vi "UMLEditor Main.vi"(1 "StartProject":string, 3 "StartTarget":string) -> ()   [LabVIEW 2012] (continued)
                              n889 = call-dynamic "translate.vi"("reference"=w2613, "dx"=w2615, "dy"=w2614, "error in (no error)"=w2617) -> ("error out"=w2616:errorcluster)  [unwired: 14 in, 1 out]
                            }
                          }
                        }
                        n890 = Bundle By Name(cluster=w2551, "state"=UMLEditor_statesType."Repaint") -> (w2561:T7)
                        n891 = Array Size(array=w2540) -> (size(s)=w2539:i32)
                        n892 = case shown="Default" w2539 {
                          tunnel: w2559 -> [w2574 w2578]
                          tunnel: [w2574 w2577] -> w2558
                          tunnel: w2553 -> [_ w2576]
                          tunnel: w2540 -> [_ w2575]
                          frame Default {
                          }
                          frame 1.. {
                            n893 = call-dynamic "layout.vi"("reference"=w2576, "LayoutNodes(Empty=All)"=w2575, "error in (no error)"=w2578) -> ("error out"=w2577:errorcluster)  [unwired: 15 in, 1 out]
                          }
                        }
                        n894 = call <resource>:"UMLEditor setDiagramInfo.vi"("error in (no error)"=w2558, "localVariablesIn"=w2561, "action"=enum16{"Name/Dir", "Unsaved", "Saved"}."Unsaved") -> ("localVariablesOut"=w2552:T7, "error out"=w2556:errorcluster)  [unwired: 2 in, 13 out]
                      }
                      frame Default {
                      }
                    }
                  }
                  frame True {
                  }
                }
              }
              frame "Shift" {
                n895 = case shown="Default" w2623 {
                  tunnel: [w2630 w2636] -> w2628
                  tunnel: w2627 -> [w2630 w2635]
                  tunnel: w2626 -> [_ w2634]
                  tunnel: w2625 -> [_ w2633]
                  tunnel: w2624 -> [_ w2632]
                  tunnel: w2622 -> [_ w2631]
                  frame "Key Repeat?" {
                  }
                  frame Default {
                    n896 = case shown="\"Class\"" w2632 {
                      tunnel: [w2637 w2651] -> w2636
                      tunnel: w2635 -> [w2637 w2644]
                      tunnel: w2634 -> [_ w2650]
                      tunnel: w2633 -> [_ w2649]
                      tunnel: w2631 -> [_ w2645]
                      frame "None", Default {
                        # "Only supported in Class Diagram for now"
                      }
                      frame "Class" {
                        n897 = Unbundle By Name(w2649) -> ("zoom"=w2652:dbl, "offset"=w2654:T12)
                        n898 = property on="Picture" class="Pict"() -> ("Mouse"=w2648:T42)  [unwired: 2 in, 2 out]
                        n899 = Unbundle By Name(w2648) -> ("Mouse Position"=w2647:cluster{"X":i32, "Y":i32})
                        n900 = Add(x=w2654, y=w2647) -> (x+y=w2653:T12)
                        n901 = Divide(x=w2653, y=w2652) -> (x/y=w2638:T12)
                        n902 = call <resource>:"UMLEditor_FindObject.vi"("FindManyEdges(False)"=TRUE, "offset"=w2638, "error in"=w2644, "graphics"=w2645, "graph"=w2650) -> ("error out"=w2643:errorcluster, "NodeFound"=w2642:bool, "node"=w2655:refnum<class "AbstractNode.lvclass">, "edge"=w2646:refnum<class "AbstractEdge.lvclass">, "Edges"=w2639:refnum<class "AbstractEdge.lvclass">[], "EdgeFound"=w2641:bool)  [unwired: 1 in]
                        n903 = case shown="False" w2642 {
                          tunnel: [w2658 w2671] -> w2651
                          tunnel: w2655 -> [w2662 w2674]
                          tunnel: w2638 -> [w2661 w2673]
                          tunnel: w2643 -> [w2660 w2672]
                          tunnel: w2641 -> [_ w2670]
                          tunnel: w2646 -> [_ w2669]
                          tunnel: w2639 -> [_ w2668]
                          frame True {
                            n904 = call-dynamic "GetContextHelpInfo.vi"("reference"=w2662, "MousePos"=w2661, "error in (no error)"=w2660) -> ("ContextHelpInfoExist"=w2656:bool, "ContextHelpInfo"=w2657:variant, "error out"=w2659:errorcluster)  [unwired: 13 in, 1 out]
                            n905 = case shown="False" w2656 {
                              tunnel: w2659 -> [w2663 w2667]
                              tunnel: [w2663 w2666] -> w2658
                              tunnel: w2657 -> [_ w2665]
                              frame False {
                              }
                              frame True {
                                n906 = local write "Help"(TRUE ("Help")) -> ()
                                n907 = call <resource>:"ContextHelp_SendMessageToPopUp.vi"("PopUpMessage"=w2665, "error in (no error)"=w2667) -> ("error out"=w2666:errorcluster)  [unwired: 1 in, 16 out]
                              }
                            }
                          }
                          frame False {
                            n908 = case shown="True" w2670 {
                              tunnel: w2674 -> [_ _]
                              tunnel: w2673 -> [_ w2684]
                              tunnel: w2672 -> [w2675 w2687]
                              tunnel: [w2675 w2688] -> w2671
                              tunnel: w2669 -> [_ w2685]
                              tunnel: w2668 -> [_ w2683]
                              frame False {
                              }
                              frame True {
                                w2680 = cluster{string, "empty picture":picture, string} {"Dependencies", "empty picture"=bytes[0], ""}
                                n909 = for {
                                tunnel: w2685 -> [_]
                                tunnel: w2684 -> [w2693]
                                shift-right: [w2694] -> w2686
                                shift-left: w2687 -> [w2695]
                                tunnel: w2683 -> [w2692] mode=indexing
                                tunnel: w2680 -> [_]
                                shift-right: [w2689] -> w2678
                                shift-left: string[] [] -> [w2691]
                                n910 = call-dynamic "GetContextHelpInfo.vi"("reference"=w2692, "MousePos"=w2693, "error in (no error)"=w2695) -> ("Rows"=w2690:string[], "error out"=w2694:errorcluster)  [unwired: 12 in, 3 out]
                                n911 = for {
                                shift-right: [w2699] -> w2689
                                shift-left: w2691 -> [w2698]
                                tunnel: w2690 -> [w2697] mode=indexing
                                n912 = Search 1D Array(1D array=w2698, element=w2697) -> (index of element=w2696:i32)  [unwired: 1 in]
                                n913 = case shown="-1" w2696 {
                                tunnel: w2698 -> [w2700 w2703]
                                tunnel: w2697 -> [_ w2702]
                                tunnel: [w2700 w2701] -> w2699
                                frame Default {
                                }
                                frame -1 {
                                n914 = Build Array (concatenate)(w2703, w2702) -> (w2701:string[])
                                }
                                }
                                }
                                }
                                n915 = Concatenate Strings("<120>", w2678) -> (w2682:string)
                                n916 = Array Size(array=w2678) -> (size(s)=w2677:i32)
                                n917 = Bundle(cluster=w2680, w2682) -> (w2679:cluster{string, "empty picture":picture, string})  [unwired: 2 out]
                                n918 = case shown="0, Default" w2677 {
                                tunnel: w2686 -> [w2704 w2708]
                                tunnel: [w2704 w2707] -> w2688
                                tunnel: w2679 -> [_ w2706]
                                frame 0, Default {
                                }
                                frame 1.. {
                                n919 = local write "Help"(TRUE ("Help")) -> ()
                                n920 = call <resource>:"ContextHelp_SendMessageToPopUp.vi"("PopUpMessage"=w2706, "error in (no error)"=w2708) -> ("error out"=w2707:errorcluster)  [unwired: 1 in, 16 out]
                                }
                                }
                              }
                            }
                          }
                        }
                      }
                    }
                  }
                }
              }
              frame "F5" {
                n921 = Bundle By Name(cluster=w2711, "state"=UMLEditor_statesType."Repaint") -> (w2710:T7)
              }
              frame "Ctrl", "Alt" {
              }
            }
            n922 = event-data() -> ()  [unwired: 1 in, 6 out]
          }
          event Application Instance Close? {
            n923 = event-data() -> ()  [unwired: 3 out]
            n924 = Bundle By Name(cluster=w2718, "state"=UMLEditor_statesType."Exit") -> (w2719:T7)
            n925 = event-data("Discard?"=TRUE) -> ()  [unwired: 1 in, 1 out]
          }
          event Panel Close? {
            w2720 = FALSE ("Sync")
            n926 = event-data() -> ()  [unwired: 4 out]
            n927 = local write "Sync"(w2720) -> ()
            n928 = Bundle By Name(cluster=w2723, "state"=UMLEditor_statesType."Exit", "Sync"=w2720) -> (w2724:T7)
            n929 = event-data("Discard?"=TRUE) -> ()  [unwired: 1 in, 1 out]
          }
          event Menu Selection (User) {
            n930 = event-data() -> ("MenuRef"=w2733:refnum<k9>, "ItemTag"=w2734:string)  [unwired: 5 out]
            n931 = case shown="\"APP_PROJECT_NEW\"" w2734 {
              selector: w2734 -> [w2747 _ _ _ _ _ _ _ _ w2839 _ _ _ _ w2873 w2880 _ _ _ _ w2985 w3045 w3054 w3069 w3085 w3108 _ _ _ _ _ _ _ _ _ _ _ _ _ _]
              tunnel: w2726 -> [w2736 w2760 w2762 w2770 w2786 w2797 w2807 w2813 w2819 w2836 w2852 w2854 w2860 w2866 w2875 w2882 w2885 w2924 w2946 w2954 w2966 w3047 w3057 w3071 w3089 w3111 w3121 w3126 w3128 w3132 w3136 w3140 w3146 w3152 w3161 w3167 w3175 w3178 w3196 w3205]
              tunnel: w2733 -> [_ _ _ _ _ _ _ _ _ w2833 _ _ _ _ _ _ _ _ _ _ _ _ w3062 w3075 _ _ _ _ _ _ _ _ _ _ _ _ _ _ _ _]
              tunnel: w2732 -> [w2748 w2759 w2761 w2767 w2791 w2802 w2804 w2808 w2823 w2830 w2851 w2856 w2862 w2868 w2874 w2884 w2887 w2920 w2950 w2952 w2991 w3049 w3061 w3074 w3088 w3100 w3119 w3123 w3127 w3129 w3133 w3137 w3144 w3150 w3160 w3165 w3174 w3179 w3192 w3206]
              tunnel: [w2748 w2758 w2761 w2763 w2787 w2798 w2804 w2808 w2822 w2841 w2851 w2856 w2862 w2868 w2874 w2884 w2886 w2923 w2950 w2952 w2988 w3049 w3055 w3066 w3087 w3096 w3119 w3123 w3127 w3129 w3133 w3137 w3144 w3150 w3160 w3165 w3173 w3179 w3181 w3206] -> w2731
              tunnel: [w2740 w2760 w2762 w2770 w2785 w2796 w2806 w2813 w2819 w2835 w2852 w2857 w2863 w2869 w2876 w2883 w2885 w2922 w2949 w2953 w2976 w3048 w3056 w3070 w3090 w3112 w3122 w3125 w3128 w3131 w3135 w3139 w3145 w3151 w3161 w3166 w3175 w3177 w3195 w3205] -> w2728
              tunnel: w2730 -> [_ _ _ _ w2790 w2801 _ _ _ _ _ _ _ _ _ _ _ _ _ _ _ _ _ _ _ w3095 _ _ _ _ _ _ _ _ _ _ _ _ w3184 _]
              tunnel: w2729 -> [_ _ _ _ _ _ _ _ _ _ _ _ _ _ _ _ _ _ _ _ _ _ _ _ _ w3094 _ _ _ _ _ _ w3143 w3149 _ w3164 _ _ _ _]
              tunnel: w2727 -> [_ _ _ _ w2783 w2794 _ _ _ _ _ _ _ _ _ _ _ _ _ _ _ _ _ _ _ _ _ _ _ _ _ _ _ _ _ _ _ _ _ _]
              frame Default {
                w2737 = FALSE ("Sync")
                n932 = String To Path(string=w2747) -> (path=w2739:path)
                n933 = Bundle By Name(cluster=w2736, "Sync"=w2737) -> (w2735:T7)
                n934 = local write "Sync"(w2737) -> ()
                n935 = File/Directory Info(path=w2739) -> (directory=w2742:bool, size=w2738:i64, error out=w2745:errorcluster)  [unwired: 1 in, 4 out]
                n936 = To Long Integer(number=w2738) -> (32bit integer=w2746:i32)
                n937 = Unbundle By Name(w2745) -> ("status"=w2743:bool)
                n938 = Greater Than 0?(x=w2746) -> (x > 0?=w2744:bool)
                n939 = Compound Arithmetic op=AND(invert w2742, w2744, invert w2743) -> (w2741:bool)
                n940 = case shown="True" w2741 {
                  tunnel: w2735 -> [w2753 w2757]
                  tunnel: [w2753 w2756] -> w2740
                  tunnel: w2739 -> [w2752 w2754]
                  frame False {
                    n941 = Strip Path(path=w2752) -> (name=w2751:string)  [unwired: 1 out]
                    n942 = Format Into String(format string="File missing\nThis file could not be located.\n%s" ("message"), w2751) -> (resulting string=w2749:string)  [unwired: 2 in, 1 out]
                    n943 = One Button Dialog(message=w2749) -> ()  [unwired: 2 out]
                  }
                  frame True {
                    n944 = Bundle By Name(cluster=w2757, "state"=UMLEditor_statesType."Open", "file"=w2754) -> (w2756:T7)
                  }
                }
              }
              frame "About" {
                n945 = call <resource>:"OpenGDSLicense_ProductInfo.vi"("error in (no error)"=w2759) -> ("error out"=w2758:errorcluster)  [unwired: 18 in]
              }
              frame "APP_PROJECT_NEW" {
                n946 = invoke class="App" method="Project.NewWithPrompts"() -> ()  [unwired: 3 in, 3 out]
              }
              frame "OpenVI" {
                n947 = call "File Dialog2"("prompt"="Select VI to open", "error in"=w2767, "pattern (all files)"="*.vi") -> ("selected path"=w2765:path, "cancelled"=w2764:bool, "error out"=w2766:errorcluster)  [unwired: 4 in, 6 out]
                n948 = case shown="False" w2764 {
                  tunnel: w2766 -> [w2773 w2781]
                  tunnel: w2765 -> [w2772 _]
                  tunnel: [w2771 w2781] -> w2763
                  frame False {
                    n949 = call <resource>:"CommonVIs_UmlOpenVIRef.vi"("error in"=w2773) -> ("error out"=w2775:errorcluster, "AppRefOut"=w2774:refnum<vi>)  [unwired: 3 in, 6 out]
                    n950 = Open VI Reference(application reference (local)=w2774, vi path=w2772, error in (no error)=w2775) -> (vi reference=w2780:refnum<vi>, error out=w2776:errorcluster)  [unwired: 3 out]
                    n951 = property class="VI"(reference=w2780, error in=w2776, "Front Panel Window:Open"=TRUE) -> (reference out=w2778:refnum<vi>, error out=w2777:errorcluster)
                    n952 = Close Reference(reference=w2778, error in (no error)=w2777) -> (error out=w2771:errorcluster)
                  }
                  frame True {
                  }
                }
              }
              frame "Undo" {
                n953 = Unbundle By Name(w2783) -> ("graphics"=w2789:refnum<class "Graphics.lvclass">, "grid"=w2788:refnum<class "Grid.lvclass">)
                n954 = Unbundle By Name(w2783) -> ("menu"=w2782:refnum<k9>)
                n955 = call <resource>:"UndoEngine.vi"("reference"=w2790, "Action"=enum16{"TakeSnapshot", "Undo", "Redo"}."Undo", "graphics"=w2789, "grid"=w2788, "error in (no error)"=w2791, "menu"=w2782) -> ("error out"=w2787:errorcluster)  [unwired: 2 in, 11 out]
                n956 = Bundle By Name(cluster=w2786, "state"=UMLEditor_statesType."Repaint") -> (w2785:T7)
              }
              frame "Redo" {
                n957 = Unbundle By Name(w2794) -> ("graphics"=w2800:refnum<class "Graphics.lvclass">, "grid"=w2799:refnum<class "Grid.lvclass">)
                n958 = Unbundle By Name(w2794) -> ("menu"=w2793:refnum<k9>)
                n959 = call <resource>:"UndoEngine.vi"("reference"=w2801, "Action"=enum16{"TakeSnapshot", "Undo", "Redo"}."Redo", "graphics"=w2800, "grid"=w2799, "error in (no error)"=w2802, "menu"=w2793) -> ("error out"=w2798:errorcluster)  [unwired: 2 in, 11 out]
                n960 = Bundle By Name(cluster=w2797, "state"=UMLEditor_statesType."Repaint") -> (w2796:T7)
              }
              frame "EnterNewLicenceKey" {
                n961 = Bundle By Name(cluster=w2807, "state"=UMLEditor_statesType."CheckLicense") -> (w2806:T7)
              }
              frame "SendComments" {
                n962 = call <resource>:"UMLEditor CommentsDialog.vi"() -> ("nameOut"=w2811:string, "commentsOut"=w2810:string, "canceled"=w2809:bool, "error out"=w2812:errorcluster)  [unwired: 1 in, 15 out]
                n963 = case shown="True" w2809 {
                  tunnel: w2812 -> [w2817 w2818]
                  tunnel: w2811 -> [w2816 _]
                  tunnel: w2810 -> [w2815 _]
                  tunnel: [w2814 w2818] -> _
                  frame False {
                    n964 = call <resource>:"UMLEditor PostComment.vi"("name"=w2816, "comment"=w2815, "error in (no error)"=w2817) -> ("error out"=w2814:errorcluster)  [unwired: 16 out]
                  }
                  frame True {
                  }
                }
              }
              frame "Help_1" {
                n965 = local read "Help"() -> (w2821:bool)
                n966 = Not(x=w2821) -> (.not. x?=w2820:bool)
                n967 = local write "Help"(w2820) -> ()
                n968 = case shown="True" w2820 {
                  tunnel: [ContextHelp_HelpTexts."None(Hide)" ("HelpText") ContextHelp_HelpTexts."Default" ("HelpText")] -> w2824
                  frame False {
                  }
                  frame True {
                  }
                }
                n969 = call <resource>:"ContextHelp_HelpTexts.vi"("HelpText (enum or string)"=w2824) -> ("HelpOut"=w2825:T57)  [unwired: 18 out]
                n970 = call <resource>:"ContextHelp_SendMessageToPopUp.vi"("PopUpMessage"=w2825, "error in (no error)"=w2823) -> ("error out"=w2822:errorcluster)  [unwired: 1 in, 16 out]
              }
              frame "Help_Class Diagram", "Help_Sequence Diagram", "Help_State Diagram", "Help_Use Case Diagram" {
                n971 = local write "Help"("Help") -> ()
                n972 = Set Menu Item Info(6:FALSE ("ToolHelp"), 7:"Show Context Help for tools" ("item tag"), 8:w2830, 11:w2833) -> (0:w2838:errorcluster)  [unwired: 4 out]
                n973 = case shown="True" "Help" {
                  tunnel: [ContextHelp_HelpTexts."None(Hide)" ("HelpText") w2846] -> w2842
                  tunnel: w2839 -> [_ w2845]
                  frame False {
                  }
                  frame True {
                    n974 = case shown="\"Help_Use Case Diagram\"" w2845 {
                      tunnel: [ContextHelp_HelpTexts."ClassDiagram_Help" ("HelpText") ContextHelp_HelpTexts."UseCaseDiagram_Help" ("HelpText") ContextHelp_HelpTexts."SequenceDiagram_Help" ("HelpText") ContextHelp_HelpTexts."StateDiagram_Help" ("HelpText")] -> w2846
                      frame "Help_Class Diagram", Default {
                      }
                      frame "Help_Use Case Diagram" {
                      }
                      frame "Help_Sequence Diagram" {
                      }
                      frame "Help_State Diagram" {
                      }
                    }
                  }
                }
                n975 = call <resource>:"ContextHelp_Memory.vi"("State"=FALSE ("ToolHelp"), "error in (no error)"=w2838, "Actio(GetStatus)n"=T27."SetToolHelp") -> ("error out"=w2831:errorcluster)  [unwired: 1 in, 15 out]
                n976 = call <resource>:"ContextHelp_HelpTexts.vi"("HelpText (enum or string)"=w2842) -> ("HelpOut"=w2843:T57)  [unwired: 18 out]
                n977 = call <resource>:"ContextHelp_SendMessageToPopUp.vi"("PopUpMessage"=w2843, "error in (no error)"=w2831) -> ("error out"=w2841:errorcluster)  [unwired: 1 in, 16 out]
                n978 = Bundle By Name(cluster=w2836, "ToolHelp"=FALSE) -> (w2835:T7)
              }
              frame "GettingStarted" {
                n979 = call <resource>:"UMLEditor GettingStartedDialog.vi"() -> ()  [unwired: 1 out]
              }
              frame "Properties" {
                w2855 = FALSE ("Sync")
                n980 = Bundle By Name(cluster=w2854, "Sync"=w2855) -> (w2853:T7)
                n981 = local write "Sync"(w2855) -> ()
                n982 = Bundle By Name(cluster=w2853, "state"=UMLEditor_statesType."EditSelected") -> (w2857:T7)
              }
              frame "Class Reversed Engineering" {
                w2861 = FALSE ("Sync")
                n983 = Bundle By Name(cluster=w2860, "Sync"=w2861) -> (w2859:T7)
                n984 = local write "Sync"(w2861) -> ()
                n985 = Bundle By Name(cluster=w2859, "state"=UMLEditor_statesType."ClassReversedEngineering") -> (w2863:T7)
              }
              frame "State Reversed Engineering" {
                w2867 = FALSE ("Sync")
                n986 = Bundle By Name(cluster=w2866, "Sync"=w2867) -> (w2865:T7)
                n987 = local write "Sync"(w2867) -> ()
                n988 = Bundle By Name(cluster=w2865, "state"=UMLEditor_statesType."StateReversedEngineering") -> (w2869:T7)
              }
              frame "Delete", "Remove package only" {
                n989 = Equal?(x=w2873, y="Remove package only") -> (x = y?=w2871:bool)
                n990 = Bundle By Name(cluster=w2875, "state"=UMLEditor_statesType."RemoveSelected", "Don'tDeleteChildren"=w2871) -> (w2876:T7)
              }
              frame "Save", "Save As" {
                n991 = Equal?(x="Save As", y=w2880) -> (x = y?=w2878:bool)
                n992 = Bundle By Name(cluster=w2882, "state"=UMLEditor_statesType."Save", "saveAs"=w2878) -> (w2883:T7)
              }
              frame "Export to XMI" {
                (unwired) T58."new or existing file" ("select mode (2)")
                n993 = call <resource>:"UMLEditor getDiagramInfo.vi"("localVariables"=w2885, "error in (no error)"=w2887) -> ("graph"=w2888:refnum<class "Graph.lvclass">, "name"=w2895:string, "diagramType"=w2889:T11, "saveDir"=w2899:path, "error out"=w2890:errorcluster)  [unwired: 13 out]
                n994 = Build Path(base path=w2899, name or relative path=w2895) -> (appended path=w2896:path)
                n995 = call <vilib>:"Get File Extension.vi"("file"=w2896) -> ("filename without extension"=w2897:string)  [unwired: 1 in, 9 out]
                n996 = Concatenate Strings(w2897, ".xmi" ("string")) -> (w2900:string)
                n997 = File Dialog(6:"*.xmi" ("pattern"), 7:"Select file name" ("prompt"), 9:w2900, 11:w2899) -> (1:w2891:bool, 2:w2892:bool, 3:w2902:path)  [unwired: 1 in, 3 out]
                n998 = case shown="True" w2892 {
                  tunnel: [w2910 w2913] -> w2901
                  tunnel: w2891 -> [w2910 _]
                  tunnel: w2902 -> [w2911 w2912]
                  tunnel: [w2911 w2912] -> _
                  frame False {
                  }
                  frame True {
                    n999 = Two Button Dialog(message="This file already exists.\nDo you want to overwrite it?", 1:"No" ("F button name (\"Cancel\")"), 2:"Yes" ("T button name (\"OK\")")) -> (T button?=w2914:bool)
                    n1000 = case shown="True" w2914 {
                      tunnel: w2912 -> [_ w2918]
                      frame False {
                      }
                      frame True {
                        n1001 = Delete(path (use dialog)=w2918) -> ()  [unwired: 1 in, 6 out]
                      }
                    }
                    n1002 = Not(x=w2914) -> (.not. x?=w2913:bool)
                  }
                }
                n1003 = case shown="False" w2901 {
                  tunnel: w2888 -> [w2908 _]
                  tunnel: w2889 -> [w2907 _]
                  tunnel: w2890 -> [w2906 w2909]
                  tunnel: w2902 -> [w2905 _]
                  tunnel: [w2903 w2909] -> w2886
                  frame False {
                    n1004 = call-dynamic "saveGraph.vi"("reference"=w2908, "filePath"=w2905, "diagramType"=w2907, "error in (no error)"=w2906, "ExportType(Normal)"=SaveTypes."XMI") -> ("error out"=w2903:errorcluster)  [unwired: 12 in, 2 out]
                  }
                  frame True {
                  }
                }
              }
              frame "Import from XMI" {
                n1005 = call "File Dialog3"("prompt"="Select XMI file to import", "error in"=w2920, "pattern (all files)"="*.xm?", "pattern label"="XMI file") -> ("selected path"=w2921:path, "exists"=w2927:bool, "cancelled"=w2926:bool, "error out"=w2919:errorcluster)  [unwired: 8 in]
                n1006 = Compound Arithmetic op=AND(w2927, invert w2926, invert w2919) -> (w2925:bool)
                n1007 = case shown="False" w2925 {
                  tunnel: w2924 -> [w2931 w2937]
                  tunnel: w2920 -> [w2932 w2936]
                  tunnel: [w2932 w2936] -> w2923
                  tunnel: [w2931 w2938] -> w2922
                  tunnel: w2921 -> [_ w2935]
                  frame False {
                  }
                  frame True {
                    w2939 = FALSE ("Sync")
                    n1008 = local write "Sync"(w2939) -> ()
                    n1009 = Path To String(path=w2935) -> (string=w2934:string)
                    n1010 = Bundle By Name(cluster=w2937, "selectedEdge"=refnum<class "AbstractEdge.lvclass"> refnum, "SelectedNodes"=refnum<class "AbstractNode.lvclass">[] [], "selcted"=UMLEditor_tooltype."None", "state"=UMLEditor_statesType."ClassReversedEngineering", "toolType"=UMLEditor_tooltype."None", "Sync"=w2939, "Action"=w2934, "XMI_Import"=TRUE ("Sync")) -> (w2938:T7)
                  }
                }
              }
              frame "Open" {
                w2947 = FALSE ("Sync")
                n1011 = Bundle By Name(cluster=w2946, "Sync"=w2947) -> (w2945:T7)
                n1012 = local write "Sync"(w2947) -> ()
                n1013 = Bundle By Name(cluster=w2945, "state"=UMLEditor_statesType."Open") -> (w2949:T7)
              }
              frame "Close" {
                w2951 = FALSE ("Sync")
                n1014 = Unbundle By Name(w2954) -> ("diagrams"=w2961:T39)
                n1015 = Array Size(array=w2961) -> (size(s)=w2960:i32)
                n1016 = Greater Than 0?(x=w2960) -> (x > 0?=w2959:bool)
                n1017 = Select(t=UMLEditor_statesType."Close" ("state"), s=w2959, f=UMLEditor_statesType."Idle" ("state")) -> (s? t:f=w2957:T8)
                n1018 = local write "Sync"(w2951) -> ()
                n1019 = Bundle By Name(cluster=w2954, "state"=w2957, "selcted"=UMLEditor_tooltype."None", "Sync"=w2951) -> (w2953:T7)
              }
              frame "Class Diagram", "Sequence Diagram", "State Diagram", "Use Case Diagram" {
                w2962 = FALSE ("Sync")
                n1020 = case shown="\"State Diagram\"" w2985 {
                  tunnel: w2991 -> [w3027 w3030 w3034 w3038]
                  tunnel: [w3026 w3028 w3032 w3036] -> w2967
                  tunnel: [w3025 w3029 w3033 w3037] -> w2963
                  tunnel: [diagramType."Class" ("diagramType") diagramType."Sequency" ("diagramType") diagramType."UseCase" ("diagramType") diagramType."State" ("diagramType")] -> w2978
                  frame "Class Diagram", Default {
                    n1021 = call <resource>:"ClassDiagramGraph_Create.vi"("error in (no error)"=w3027) -> ("reference out"=w3026:refnum<class "ClassDiagramGraph.lvclass">, "error out"=w3025:errorcluster)  [unwired: 2 in, 15 out]
                  }
                  frame "Sequence Diagram" {
                    n1022 = call <resource>:"SequenceDiagramGraph_Create.vi"("error in (no error)"=w3030) -> ("reference out"=w3028:refnum<class "SequenceDiagramGraph.lvclass">, "error out"=w3029:errorcluster)  [unwired: 2 in, 15 out]
                  }
                  frame "Use Case Diagram" {
                    n1023 = call <resource>:"UseCaseDiagramGraph_Create.vi"("error in (no error)"=w3034) -> ("reference out"=w3032:refnum<class "UseCaseDiagramGraph.lvclass">, "error out"=w3033:errorcluster)  [unwired: 2 in, 15 out]
                  }
                  frame "State Diagram" {
                    n1024 = call <resource>:"StateDiagramGraph_Create.vi"("error in (no error)"=w3038) -> ("reference out"=w3036:refnum<class "StateDiagramGraph.lvclass">, "error out"=w3037:errorcluster)  [unwired: 3 in, 14 out]
                  }
                }
                n1025 = property on="toolTab" class="TabCtl (strict)"("Disabled"=u8 0) -> ()  [unwired: 2 in, 2 out]
                n1026 = local write "Diagram"(0) -> ()
                n1027 = property on="Picture" class="Pict"("Visible"=TRUE) -> ()  [unwired: 2 in, 2 out]
                n1028 = Unbundle By Name(w2966) -> ("diagrams"=w2996:T39)
                n1029 = Unbundle By Name(w2966) -> ("menu"=w2965:refnum<k9>)
                n1030 = for {
                  tunnel: w2996 -> [w3043] mode=indexing
                  tunnel: "Untitled %d" -> [w3041]
                  tunnel: [w3040] -> w2994 mode=indexing
                  n1031 = Unbundle By Name(w3043) -> ("name"=w3042:string)
                  n1032 = Scan From String(format string=w3041, input string=w3042) -> (output 1=w3040:i32)  [unwired: 2 in, 4 out]
                }
                n1033 = call <resource>:"UndoEngine.vi"("reference"=w2967, "Action"=enum16{"TakeSnapshot", "Undo", "Redo"}."TakeSnapshot", "Reset"=TRUE, "error in (no error)"=w2963, "menu"=w2965) -> ("error out"=w2964:errorcluster)  [unwired: 3 in, 11 out]
                n1034 = local read "Help"() -> (w2979:bool)
                n1035 = Array Max & Min(array=w2994) -> (max value=w2993:i32)  [unwired: 3 out]
                n1036 = case shown="True" w2979 {
                  tunnel: w2978 -> [_ w3000]
                  frame False {
                  }
                  frame True {
                    n1037 = case shown="\"Class\", Default" w3000 {
                      tunnel: [ContextHelp_HelpTexts."ClassDiagram_Help" ("HelpText") ContextHelp_HelpTexts."UseCaseDiagram_Help" ("HelpText") ContextHelp_HelpTexts."SequenceDiagram_Help" ("HelpText") ContextHelp_HelpTexts."StateDiagram_Help" ("HelpText")] -> w2998
                      frame "Class", Default {
                      }
                      frame "UseCase" {
                      }
                      frame "Sequency" {
                      }
                      frame "State" {
                      }
                    }
                    n1038 = call <resource>:"ContextHelp_HelpTexts.vi"("HelpText (enum or string)"=w2998) -> ("HelpOut"=w2999:T57)  [unwired: 18 out]
                    n1039 = call <resource>:"ContextHelp_SendMessageToPopUp.vi"("PopUpMessage"=w2999) -> ()  [unwired: 2 in, 17 out]
                  }
                }
                n1040 = Increment(x=w2993) -> (x+1=w2990:i32)
                n1041 = call <resource>:"UMLEditor UpdatesToolbuttons.vi"() -> ()  [unwired: 6 in, 14 out]
                n1042 = Format Into String(format string="Untitled %d", w2990) -> (resulting string=w2982:string)  [unwired: 2 in, 1 out]
                n1043 = call <resource>:"UMLEditor addDiagram.vi"("graph"=w2967, "diagramType"=w2978, "name"=w2982, "saveDir"=path "", "unsaved(False)"=FALSE, "error in (no error)"=w2964, "localVariablesIn"=w2966) -> ("localVariablesOut"=w2983:T7, "error out"=w2987:errorcluster)  [unwired: 11 out]
                n1044 = property on="Diagram" class="Ring (strict)"("Tip Strip"=w2982) -> ()  [unwired: 2 in, 2 out]
                n1045 = case shown="\"Sequency\"" w2978 {
                  tunnel: w2983 -> [w3006 w3010 w3014 w3019 w3023]
                  tunnel: [w3005 w3009 w3013 w3018 w3022] -> w2975
                  frame "None" {
                    n1046 = Bundle By Name(cluster=w3006, "tool"=UMLEditor_toolsType."CD_Select") -> (w3005:T7)
                  }
                  frame "Sequency" {
                    n1047 = Bundle By Name(cluster=w3010, "tool"=UMLEditor_toolsType."SQD_Select") -> (w3009:T7)
                    n1048 = property on="toolTab" class="TabCtl (strict)"("Value"=enum32{"Class", "Sequence", "UseCase"}."Sequence" ("toolTab")) -> ()  [unwired: 2 in, 2 out]
                  }
                  frame "UseCase" {
                    n1049 = Bundle By Name(cluster=w3014, "tool"=UMLEditor_toolsType."UD_Select") -> (w3013:T7)
                    n1050 = property on="toolTab" class="TabCtl (strict)"("Value"=enum32{"Class", "Sequence", "UseCase"}."UseCase" ("toolTab")) -> ()  [unwired: 2 in, 2 out]
                  }
                  frame "State" {
                    n1051 = Bundle By Name(cluster=w3019, "tool"=UMLEditor_toolsType."STD_Select") -> (w3018:T7)
                    n1052 = property on="toolTab" class="TabCtl (strict)"("Value"=enum32{"Class", "Sequence", "UseCase", "State"}."State" ("toolTab")) -> ()  [unwired: 2 in, 2 out]
                  }
                  frame "Class", Default {
                    n1053 = Bundle By Name(cluster=w3023, "tool"=UMLEditor_toolsType."CD_Select") -> (w3022:T7)
                    n1054 = property on="toolTab" class="TabCtl (strict)"("Value"=enum32{"Class", "Sequence", "UseCase"}."Class" ("toolTab")) -> ()  [unwired: 2 in, 2 out]
                  }
                }
                n1055 = Unbundle By Name(w2966) -> ("menu"=w2977:refnum<k9>)
                n1056 = Bundle By Name(cluster=w2975, "selectedEdge"=refnum<class "AbstractEdge.lvclass"> refnum, "SelectedNodes"=refnum<class "AbstractNode.lvclass">[] [], "selcted"=UMLEditor_tooltype."None", "state"=UMLEditor_statesType."Repaint", "toolType"=UMLEditor_tooltype."None", "Sync"=w2962) -> (w2976:T7)
                n1057 = local write "Sync"(w2962) -> ()
                n1058 = call <resource>:"UMLEditor menuUpdates.vi"("menu"=w2977, "menuAction"=UMLEditor_MenuActionType."EnableSave", "error in (no error)"=w2987) -> ("error out"=w2988:errorcluster)  [unwired: 3 in, 13 out]
              }
              frame "Print", "jpg", "png" {
                n1059 = case shown="\"Print\", Default" w3045 {
                  tunnel: [UMLEditor_ExportType."Printer" ("exportype") UMLEditor_ExportType."png" ("exportype") UMLEditor_ExportType."jpg" ("exportype")] -> w3044
                  frame "Print", Default {
                  }
                  frame "png" {
                  }
                  frame "jpg" {
                  }
                }
                n1060 = Bundle By Name(cluster=w3047, "state"=UMLEditor_statesType."Export", "exportype"=w3044) -> (w3048:T7)
              }
              frame "Hide Grid" {
                n1061 = Get Menu Item Info(7:w3054, 8:w3061, 11:w3062) -> (0:w3060:errorcluster, 3:w3053:refnum<k9>, 4:w3059:bool)  [unwired: 4 out]
                n1062 = Not(x=w3059) -> (.not. x?=w3058:bool)
                n1063 = Set Menu Item Info(6:w3058, 7:w3054, 8:w3060, 11:w3053) -> (0:w3055:errorcluster)  [unwired: 4 out]
                n1064 = Bundle By Name(cluster=w3057, "state"=UMLEditor_statesType."Repaint", "hideGrid"=w3058) -> (w3056:T7)
              }
              frame "Show Context Help for tools" {
                n1065 = Get Menu Item Info(7:w3069, 8:w3074, 11:w3075) -> (0:w3073:errorcluster, 3:w3068:refnum<k9>, 4:w3072:bool)  [unwired: 4 out]
                n1066 = Not(x=w3072) -> (.not. x?=w3064:bool)
                n1067 = Set Menu Item Info(6:w3064, 7:w3069, 8:w3073, 11:w3068) -> (0:w3067:errorcluster)  [unwired: 4 out]
                n1068 = call <resource>:"ContextHelp_Memory.vi"("State"=w3064, "error in (no error)"=w3067, "Actio(GetStatus)n"=T27."SetToolHelp") -> ("error out"=w3066:errorcluster)  [unwired: 1 in, 15 out]
                n1069 = Bundle By Name(cluster=w3071, "ToolHelp"=w3064) -> (w3070:T7)
              }
              frame "Zoom In", "Zoom Out" {
                w3080 = 1.5 ("x")
                n1070 = Unbundle By Name(w3089) -> ("graphics"=w3091:refnum<class "Graphics.lvclass">, "zoom"=w3086:dbl)
                n1071 = Equal?(x=w3085, y="Zoom In") -> (x = y?=w3082:bool)
                n1072 = Square Root(x=w3080) -> ()  [unwired: 1 out]
                n1073 = Multiply(x=w3086, y=w3080) -> (x*y=w3083:dbl)
                n1074 = Divide(x=w3086, y=w3080) -> (x/y=w3081:dbl)
                n1075 = Select(t=w3083, s=w3082, f=w3081) -> (s? t:f=w3077:dbl)
                n1076 = In Range and Coerce(upper limit=5.0625, x=w3077, lower limit=0.197530864) -> (coerced(x)=w3076:dbl)  [unwired: 1 out]
                n1077 = call <resource>:"scale.vi"("reference"=w3091, "scaleX"=w3076, "scaleY"=w3076, "error in (no error)"=w3088) -> ("error out"=w3087:errorcluster)  [unwired: 15 out]
                n1078 = Bundle By Name(cluster=w3089, "zoom"=w3076, "state"=UMLEditor_statesType."Repaint") -> (w3090:T7)
              }
              frame "Larger Grid", "Smaller Grid" {
                n1079 = Unbundle By Name(w3111) -> ("grid"=w3099:refnum<class "Grid.lvclass">, "gridSize"=w3110:dbl)
                n1080 = Equal?(x=w3108, y="Larger Grid") -> (x = y?=w3105:bool)
                n1081 = Square Root(x=2.0) -> (sqrt(x)=w3109:dbl)
                n1082 = Multiply(x=w3110, y=w3109) -> (x*y=w3106:dbl)
                n1083 = Divide(x=w3110, y=w3109) -> (x/y=w3104:dbl)
                n1084 = call <resource>:"ForceUpdate.vi"("Set"=TRUE) -> ()  [unwired: 18 in, 1 out]
                n1085 = Select(t=w3106, s=w3105, f=w3104) -> (s? t:f=w3103:dbl)
                n1086 = In Range and Coerce(upper limit=100.0, x=w3103, lower limit=4.0) -> (coerced(x)=w3098:dbl)  [unwired: 1 out]
                n1087 = call <resource>:"setGrid.vi"("reference"=w3099, "gridX"=w3098, "gridY"=w3098, "error in (no error)"=w3100) -> ("error out"=w3097:errorcluster)  [unwired: 15 out]
                n1088 = case shown="Default" w3094 {
                  tunnel: w3097 -> [w3117 w3118]
                  tunnel: [w3116 w3118] -> w3096
                  tunnel: w3095 -> [w3115 _]
                  frame Default {
                    n1089 = call-dynamic "layout.vi"("reference"=w3115, "error in (no error)"=w3117) -> ("error out"=w3116:errorcluster)  [unwired: 16 in, 1 out]
                  }
                  frame "None" {
                  }
                }
                n1090 = Bundle By Name(cluster=w3111, "gridSize"=w3098, "state"=UMLEditor_statesType."Repaint") -> (w3112:T7)
              }
              frame "Exit" {
                n1091 = Bundle By Name(cluster=w3121, "state"=UMLEditor_statesType."Exit") -> (w3122:T7)
              }
              frame "createScript" {
                n1092 = Bundle By Name(cluster=w3126, "state"=UMLEditor_statesType."CreateScript") -> (w3125:T7)
              }
              frame "Open GOOP Wizard" {
                n1093 = call <resource>:"UMLEditor SendMessageToWizard.vi"("error in (no error)"=w3127) -> ()  [unwired: 3 in, 16 out]
              }
              frame "executeScript" {
                n1094 = Bundle By Name(cluster=w3132, "state"=UMLEditor_statesType."ExecuteScript") -> (w3131:T7)
              }
              frame "Copy Selected Nodes" {
                n1095 = Bundle By Name(cluster=w3136, "state"=UMLEditor_statesType."Copy") -> (w3135:T7)
              }
              frame "Paste Nodes" {
                n1096 = Bundle By Name(cluster=w3140, "state"=UMLEditor_statesType."Paste") -> (w3139:T7)
              }
              frame "AutoPlace" {
                n1097 = Not Equal?(x=diagramType."Class", y=w3143) -> ()  [unwired: 1 out]
                n1098 = Bundle By Name(cluster=w3146, "state"=UMLEditor_statesType."AutoPlace") -> (w3145:T7)
              }
              frame "Synchronize All" {
                n1099 = Not Equal?(x=diagramType."Class", y=w3149) -> (x != y?=w3147:bool)
                n1100 = case shown="False" w3147 {
                  tunnel: w3152 -> [w3155 w3157]
                  tunnel: [w3154 w3157] -> w3151
                  frame False {
                    n1101 = Bundle By Name(cluster=w3155, "state"=UMLEditor_statesType."SyncAll") -> (w3154:T7)
                  }
                  frame True {
                    n1102 = One Button Dialog(message="This is only valid for Class Diagrams") -> ()  [unwired: 2 out]
                  }
                }
              }
              frame "ToggleSync" {
                n1103 = property on="Sync" class="Bool (strict)"() -> ("Value"=w3158:bool)  [unwired: 2 in, 2 out]
                n1104 = Not(x=w3158) -> (.not. x?=w3159:bool)
                n1105 = property on="Sync" class="Bool (strict)"("Val(Sgnl)"=w3159) -> ()  [unwired: 2 in, 2 out]
              }
              frame "StraightenAssociations" {
                n1106 = Not Equal?(x=diagramType."Class", y=w3164) -> (x != y?=w3162:bool)
                n1107 = case shown="False" w3162 {
                  tunnel: w3167 -> [w3170 w3172]
                  tunnel: [w3169 w3172] -> w3166
                  frame False {
                    n1108 = Bundle By Name(cluster=w3170, "state"=UMLEditor_statesType."StraightenAssociation") -> (w3169:T7)
                  }
                  frame True {
                    n1109 = One Button Dialog(message="This is only valid for Class Diagrams") -> ()  [unwired: 2 out]
                  }
                }
              }
              frame "Revision history" {
                n1110 = call <resource>:"UMLEditor RevisionHistory.vi"("localVariables"=w3175, "error in (no error)"=w3174) -> ("error out"=w3173:errorcluster)  [unwired: 17 out]
              }
              frame "PlugInRev" {
                n1111 = Bundle By Name(cluster=w3178, "state"=UMLEditor_statesType."PlugInReverseEngineering") -> (w3177:T7)
              }
              frame "Options" {
                n1112 = call <resource>:"GetUndoOption.vi"("error in (no error)"=w3192) -> ("UndoSize"=w3189:i32, "error out"=w3191:errorcluster)  [unwired: 17 out]
                n1113 = call <resource>:"UMLEditor_OptionsDialog.vi"("localVariables"=w3196, "error in (no error)"=w3191) -> ("error out"=w3190:errorcluster)  [unwired: 1 in, 16 out]
                n1114 = call <resource>:"GetUndoOption.vi"("error in (no error)"=w3190) -> ("UndoSize"=w3183:i32, "error out"=w3187:errorcluster)  [unwired: 17 out]
                n1115 = Unbundle By Name(w3196) -> ("menu"=w3185:refnum<k9>)
                n1116 = Not Equal?(x=w3183, y=w3189) -> (x != y?=w3188:bool)
                n1117 = case shown="True" w3188 {
                  tunnel: w3187 -> [w3197 w3204]
                  tunnel: [w3197 w3203] -> w3186
                  tunnel: w3185 -> [_ w3200]
                  tunnel: w3184 -> [_ w3199]
                  tunnel: w3183 -> [_ w3198]
                  frame False {
                  }
                  frame True {
                    n1118 = call <resource>:"UndoEngine.vi"("reference"=w3199, "Action"=enum16{"TakeSnapshot", "Undo", "Redo"}."TakeSnapshot", "Reset"=TRUE, "error in (no error)"=w3204, "menu"=w3200, "UndoLevels(ignoredIfNotWired)"=w3198) -> ("error out"=w3203:errorcluster)  [unwired: 2 in, 11 out]
                  }
                }
                n1119 = call <resource>:"UMLEditor AddToolsMenuItems.vi"("menu"=w3185, "GoopWizExists"=FALSE, "error in (no error)"=w3186) -> ("error out"=w3182:errorcluster)  [unwired: 1 in, 15 out]
                n1120 = call <resource>:"GetSyncOption.vi"("error in (no error)"=w3182) -> ("SyncTime(s)"=w3180:i32, "error out"=w3181:errorcluster)  [unwired: 16 in, 1 out]
                n1121 = Bundle By Name(cluster=w3196, "state"=UMLEditor_statesType."Repaint", "SyncTime"=w3180) -> (w3195:T7)
              }
              frame "ShowTips" {
                n1122 = call <resource>:"ShowToolTips.vi"() -> ()  [unwired: 1 in, 19 out]
              }
            }
          }
          event "open": Value Change {
            n1123 = event-data() -> ()  [unwired: 6 out]
            n1124 = Bundle By Name(cluster=w3208, "state"=UMLEditor_statesType."Open") -> (w3209:T7)
          }
          event "Sync": Value Change {
            n1125 = event-data() -> ()  [unwired: 2 out]
            n1126 = case shown="False" "Sync" {
              selector: "Sync" -> [_ w3218]
              tunnel: [FALSE w3220] -> w3211
              tunnel: w3213 -> [_ w3219]
              frame False {
                n1127 = local write "StatusBar"("" ("StatusBar")) -> ()
              }
              frame True {
                n1128 = call <resource>:"UMLEditor getDiagramInfo.vi"("localVariables"=w3219) -> ("graph"=w3221:refnum<class "Graph.lvclass">, "diagramType"=w3222:T11)  [unwired: 1 in, 16 out]
                n1129 = case shown="\"Class\"" w3222 {
                  tunnel: w3218 -> [_ _]
                  tunnel: w3221 -> [_ w3232]
                  tunnel: [FALSE w3230] -> w3220
                  frame "None", Default {
                    n1130 = One Button Dialog(message="Only class diagrams can have auto synchronization turn on.") -> ()  [unwired: 1 in, 1 out]
                  }
                  frame "Class" {
                    n1131 = call-dynamic "getNodes.vi"("reference"=w3232) -> ("nodes"=w3229:refnum<class "AbstractNode.lvclass">[])  [unwired: 16 in, 2 out]
                    n1132 = for {
                      tunnel: w3229 -> [w3239] mode=indexing
                      tunnel: [w3235] -> w3231
                      stop <- w3235 continue-if-true
                      w3238 = refnum<class "ClassNode.lvclass"> refnum  # ClassNode.lvclass
                      n1133 = To More Specific Class(target class=w3238, reference=w3239) -> (specific class reference=w3237:refnum<class "ClassNode.lvclass">, error out=w3236:errorcluster)  [unwired: 1 in]
                      n1134 = case shown="No Error" w3236 {
                        selector: w3236 -> [w3245 w3247]
                        tunnel: w3237 -> [w3246 _]
                        tunnel: [w3241 w3247] -> w3235
                        frame No Error {
                          n1135 = call-dynamic "getClassInfo.vi"("reference"=w3246, "error in (no error)"=w3245) -> ("className"=w3242:string)  [unwired: 8 in, 9 out]
                          n1136 = Format Into String(format string="%s.lvclass:%s.ctl", w3242, w3242) -> (resulting string=w3243:string)  [unwired: 2 in, 1 out]
                          n1137 = call <resource>:"CommonVIs_UmlOpenVIRef.vi"("ViPath/ViName"=w3243) -> ("error out"=w3241:errorcluster, "vi reference"=w3240:refnum<vi>)  [unwired: 3 in, 6 out]
                          n1138 = Close Reference(reference=w3240) -> ()  [unwired: 1 in, 1 out]
                        }
                        frame Error {
                        }
                      }
                    }
                    n1139 = Array Size(array=w3229) -> (size(s)=w3228:i32)
                    n1140 = Equal To 0?(x=w3228) -> (x = 0?=w3226:bool)
                    n1141 = Unbundle(w3231) -> ("status"=w3227:bool)  [unwired: 2 out]
                    n1142 = Or(x=w3227, y=w3226) -> (x .or. y?=w3225:bool)
                    n1143 = case shown="True" w3225 {
                      tunnel: [TRUE _] -> w3230
                      frame False {
                      }
                      frame True {
                        n1144 = One Button Dialog(message="Synchronization can't be turned on for this diagram. Make sure at least one class have a class path defined and that the classes are in memory.") -> ()  [unwired: 1 in, 1 out]
                      }
                    }
                  }
                }
              }
            }
            n1145 = Bundle By Name(cluster=w3213, "ForceSyncNow"=w3211, "Sync"=w3211) -> (w3214:T7)
            n1146 = local write "Sync"(w3211) -> ()
          }
          event "close": Value Change {
            n1147 = event-data() -> ()  [unwired: 6 out]
            n1148 = Unbundle By Name(w3256) -> ("diagrams"=w3255:T39)
            n1149 = Array Size(array=w3255) -> (size(s)=w3254:i32)
            n1150 = Greater Than 0?(x=w3254) -> (x > 0?=w3253:bool)
            n1151 = Select(t=UMLEditor_statesType."Close" ("state"), s=w3253, f=UMLEditor_statesType."Idle" ("state")) -> (s? t:f=w3251:T8)
            n1152 = Bundle By Name(cluster=w3256, "state"=w3251, "selcted"=UMLEditor_tooltype."None") -> (w3257:T7)
          }
          event "Diagram": Value Change {
            n1153 = event-data() -> ()  [unwired: 2 out]
            n1154 = call <resource>:"UMLEditor UpdatesToolbuttons.vi"() -> ()  [unwired: 6 in, 14 out]
            n1155 = Bundle By Name(cluster=w3279, "state"=UMLEditor_statesType."Repaint", "diagramIndex"="Diagram", "toolType"=UMLEditor_tooltype."None", "selectedEdge"=refnum<class "AbstractEdge.lvclass"> refnum, "SelectedNodes"=refnum<class "AbstractNode.lvclass">[] []) -> (w3259:T7)
            n1156 = Unbundle By Name(w3259) -> ("menu"=w3258:refnum<k9>)
            n1157 = call <resource>:"UMLEditor getDiagramInfo.vi"("localVariables"=w3259, "error in (no error)"=w3276) -> ("graph"=w3262:refnum<class "Graph.lvclass">, "name"=w3267:string, "diagramType"=w3275:T11, "saveDir"=w3270:path, "error out"=w3261:errorcluster)  [unwired: 13 out]
            n1158 = case shown="\"Class\", Default" w3275 {
              tunnel: w3259 -> [w3284 w3288 w3292 w3296 w3301]
              tunnel: [w3283 w3287 w3291 w3295 w3300] -> w3274
              frame "None" {
                n1159 = property on="toolTab" class="TabCtl (strict)"("Disabled"=u8 2) -> ()  [unwired: 2 in, 2 out]
                n1160 = Bundle By Name(cluster=w3284, "tool"=UMLEditor_toolsType."CD_Select") -> (w3283:T7)
              }
              frame "Sequency" {
                n1161 = property on="toolTab" class="TabCtl (strict)"("Value"=enum32{"Class", "Sequence", "UseCase"}."Sequence" ("toolTab")) -> ()  [unwired: 2 in, 2 out]
                n1162 = Bundle By Name(cluster=w3288, "tool"=UMLEditor_toolsType."SQD_Select") -> (w3287:T7)
              }
              frame "State" {
                n1163 = Bundle By Name(cluster=w3292, "tool"=UMLEditor_toolsType."STD_Select") -> (w3291:T7)
                n1164 = property on="toolTab" class="TabCtl (strict)"("Value"=enum32{"Class", "Sequence", "UseCase", "State"}."State" ("toolTab")) -> ()  [unwired: 2 in, 2 out]
              }
              frame "UseCase" {
                n1165 = property on="toolTab" class="TabCtl (strict)"("Value"=enum32{"Class", "Sequence", "UseCase"}."UseCase" ("toolTab")) -> ()  [unwired: 2 in, 2 out]
                n1166 = Bundle By Name(cluster=w3296, "tool"=UMLEditor_toolsType."UD_Select") -> (w3295:T7)
              }
              frame "Class", Default {
                n1167 = property on="toolTab" class="TabCtl (strict)"("Value"=enum32{"Class", "Sequence", "UseCase"}."Class" ("toolTab")) -> ()  [unwired: 2 in, 2 out]
                n1168 = Bundle By Name(cluster=w3301, "tool"=UMLEditor_toolsType."CD_Select") -> (w3300:T7)
              }
            }
            n1169 = Empty String/Path?(string/path=w3270) -> (empty?=w3269:bool)
            n1170 = Build Path(base path=w3270, name or relative path=w3267) -> (appended path=w3272:path)
            n1171 = call <resource>:"UndoEngine.vi"("reference"=w3262, "Action"=enum16{"TakeSnapshot", "Undo", "Redo"}."TakeSnapshot", "Reset"=TRUE, "error in (no error)"=w3261, "menu"=w3258) -> ("error out"=w3260:errorcluster)  [unwired: 3 in, 11 out]
            n1172 = Path To String(path=w3272) -> (string=w3271:string)
            n1173 = case shown="False" w3269 {
              tunnel: w3271 -> [w3280 _]
              tunnel: [w3280 w3281] -> w3268
              tunnel: w3267 -> [_ w3281]
              frame False {
              }
              frame True {
              }
            }
            n1174 = property on="Diagram" class="Ring (strict)"("Tip Strip"=w3268) -> ()  [unwired: 2 in, 2 out]
          }
          event Panel Resize {
            w3302 = FALSE ("Sync")
            n1175 = event-data() -> ()  [unwired: 9 out]
            n1176 = local write "Sync"(w3302) -> ()
            n1177 = Bundle By Name(cluster=w3305, "ResizePanelInProgress"=TRUE, "Sync"=w3302) -> (w3304:T7)
          }
          event "Picture": Mouse Leave {
            n1178 = event-data() -> ()  [unwired: 5 out]
            n1179 = Unbundle By Name(w3313) -> ("butDwn"=w3312:bool)
            n1180 = call-poly <vilib>:"Set Cursor.vi"("VI reference (current VI)"=w3307, "icon"=u16 0) -> ()  [unwired: 1 in, 9 out]
            n1181 = Select(t=UMLEditor_statesType."Repaint" ("state"), s=w3312, f=UMLEditor_statesType."Idle" ("state")) -> (s? t:f=w3311:T8)
            n1182 = Bundle By Name(cluster=w3313, "state"=w3311) -> (w3314:T7)
          }
          event "Picture": Mouse Enter {
            n1183 = event-data() -> ()  [unwired: 5 out]
            n1184 = call-poly <vilib>:"Set Cursor.vi"("VI reference (current VI)"=w3316, "icon"=u16 1) -> ()  [unwired: 1 in, 9 out]
          }
          event "Help": Value Change {
            n1185 = event-data() -> ()  [unwired: 7 out]
            n1186 = case shown="True" "Help" {
              tunnel: [ContextHelp_HelpTexts."None(Hide)" ("HelpText") ContextHelp_HelpTexts."Default" ("HelpText")] -> w3322
              frame False {
              }
              frame True {
              }
            }
            n1187 = call <resource>:"ContextHelp_HelpTexts.vi"("HelpText (enum or string)"=w3322) -> ("HelpOut"=w3325:T57)  [unwired: 18 out]
            n1188 = call <resource>:"ContextHelp_SendMessageToPopUp.vi"("PopUpMessage"=w3325, "error in (no error)"=w3324) -> ("error out"=w3323:errorcluster)  [unwired: 1 in, 16 out]
          }
          event "Help": Mouse Enter {
            n1189 = event-data() -> ()  [unwired: 5 out]
            n1190 = Unbundle By Name(w3331) -> ("ToolHelp"=w3330:bool)
            n1191 = local read "Help"() -> (w3329:bool)
            n1192 = And(x=w3330, y=w3329) -> (x .and. y?=w3328:bool)
            n1193 = case shown="True" w3328 {
              tunnel: w3333 -> [w3334 w3337]
              tunnel: [w3334 w3336] -> w3332
              frame False {
              }
              frame True {
                n1194 = call <resource>:"ContextHelp_HelpTexts.vi"("HelpText (enum or string)"=ContextHelp_HelpTexts."Help" ("HelpText")) -> ("HelpOut"=w3338:T57)  [unwired: 18 out]
                n1195 = call <resource>:"ContextHelp_SendMessageToPopUp.vi"("PopUpMessage"=w3338, "error in (no error)"=w3337) -> ("error out"=w3336:errorcluster)  [unwired: 1 in, 16 out]
              }
            }
          }
          event Mouse Enter {
            n1196 = event-data() -> ()  [unwired: 2 out]
            n1197 = Unbundle By Name(w3342) -> ("ToolHelp"=w3341:bool)
            n1198 = local read "Help"() -> (w3340:bool)
            n1199 = And(x=w3341, y=w3340) -> (x .and. y?=w3339:bool)
            n1200 = case shown="True" w3339 {
              tunnel: w3344 -> [w3345 w3347]
              tunnel: [w3345 w3346] -> w3343
              tunnel: w3342 -> [_ _]
              frame False {
              }
              frame True {
                n1201 = call <resource>:"ContextHelp_HelpTexts.vi"("HelpText (enum or string)"=ContextHelp_HelpTexts."BSelect" ("HelpText")) -> ("HelpOut"=w3349:T57)  [unwired: 18 out]
                n1202 = call <resource>:"ContextHelp_SendMessageToPopUp.vi"("PopUpMessage"=w3349, "error in (no error)"=w3347) -> ("error out"=w3346:errorcluster)  [unwired: 1 in, 16 out]
              }
            }
          }
          event "Diagram": Mouse Enter {
            n1203 = event-data() -> ()  [unwired: 3 out]
            n1204 = Unbundle By Name(w3354) -> ("ToolHelp"=w3353:bool)
            n1205 = local read "Help"() -> (w3352:bool)
            n1206 = And(x=w3353, y=w3352) -> (x .and. y?=w3351:bool)
            n1207 = case shown="False" w3351 {
              tunnel: w3356 -> [w3357 w3361]
              tunnel: [w3357 w3360] -> w3355
              tunnel: w3354 -> [_ _]
              tunnel: w3350 -> [_ w3359]
              frame False {
              }
              frame True {
                n1208 = case shown="\"UseCase\"" w3359 {
                  tunnel: [ContextHelp_HelpTexts."Default" ("HelpText") ContextHelp_HelpTexts."ClassDiagram_Help" ("HelpText") ContextHelp_HelpTexts."SequenceDiagram_Help" ("HelpText") ContextHelp_HelpTexts."UseCaseDiagram_Help" ("HelpText") ContextHelp_HelpTexts."StateDiagram_Help" ("HelpText")] -> w3358
                  frame "None", Default {
                  }
                  frame "Class" {
                  }
                  frame "Sequency" {
                  }
                  frame "UseCase" {
                  }
                  frame "State" {
                  }
                }
                n1209 = call <resource>:"ContextHelp_HelpTexts.vi"("HelpText (enum or string)"=w3358) -> ("HelpOut"=w3362:T57)  [unwired: 18 out]
                n1210 = call <resource>:"ContextHelp_SendMessageToPopUp.vi"("PopUpMessage"=w3362, "error in (no error)"=w3361) -> ("error out"=w3360:errorcluster)  [unwired: 1 in, 16 out]
              }
            }
          }
          event Mouse Enter {
